vi "Valve Timer FGV.vi"(7 "Valve Timer Enum":T1, 8 "error in (no error)":errorcluster, 11 "Duration(min)":dbl) -> (0 "error out":errorcluster, 2 "Switch Valve":bool, 3 "Count Down [s]":dbl)   [LabVIEW 2020]
uses:
  controls/Valve Timer FGV.ctl
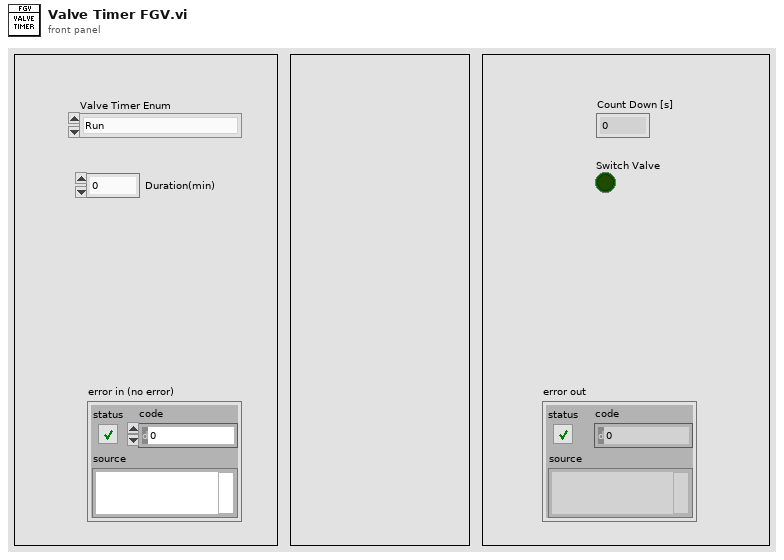
[diagram p1: front panel]
types:
  T1 = typedef "Valve Timer FGV.ctl" = enum16{"Run", "Check", "Stop"}
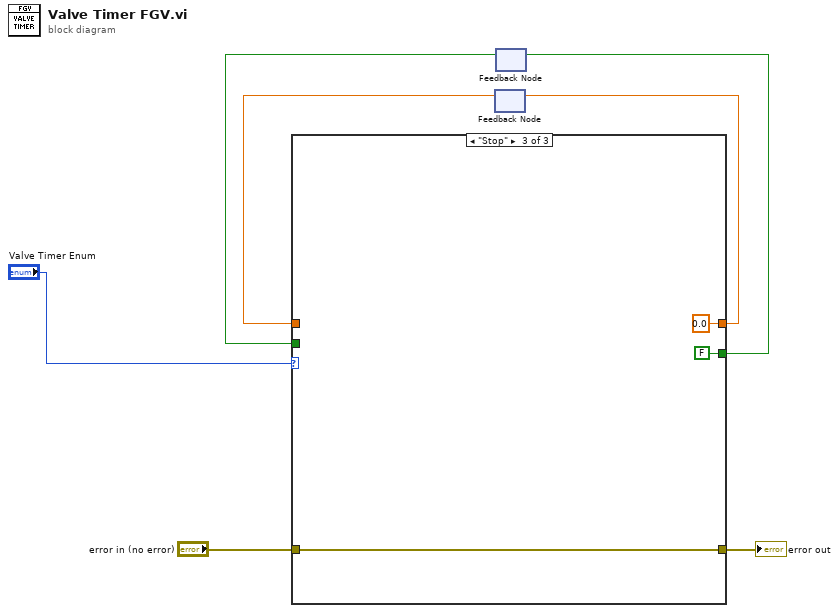
[diagram p0: block diagram]
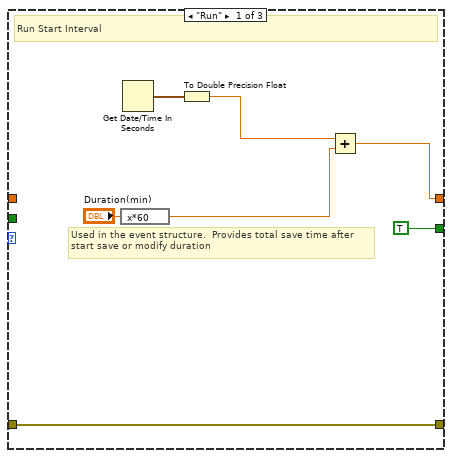
[diagram p2: hidden frame]
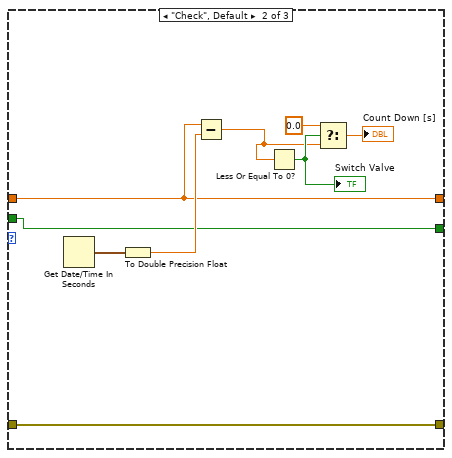
[diagram p3: hidden frame]
diagram:
  n1 = feedback #1() -> (w4:dbl)  [unwired: 1 in]
  n2 = feedback #2() -> (w1:bool)  [unwired: 1 in]
  n3 = case shown="\"Stop\"" "Valve Timer Enum" {
    tunnel: "error in (no error)" -> [w14 w23 w26]
    tunnel: [w14 w23 w26] -> w6
    tunnel: [w10 w20 0.0] -> w5
    tunnel: w4 -> [_ w20 _]
    tunnel: [TRUE w15 FALSE] -> w2
    tunnel: w1 -> [_ w15 _]
    frame "Run" {
      # "Used in the event structure.  Provides total save time after\nstart save or modify duration"
      # "Run Start Interval"
      n4 = expression code="x*60"("Duration(min)") -> (w9:dbl)
      n5 = Get Date/Time In Seconds() -> (seconds since 1Jan1904=w13:timestamp)
      n6 = To Double Precision Float(number=w13) -> (double precision float=w11:dbl)
      n7 = Add(x=w11, y=w9) -> (x+y=w10:dbl)
    }
    frame "Check", Default {
      n8 = Get Date/Time In Seconds() -> (seconds since 1Jan1904=w22:timestamp)
      n9 = To Double Precision Float(number=w22) -> (double precision float=w21:dbl)
      n10 = Subtract(x=w20, y=w21) -> (x-y=w17:dbl)
      n11 = Less Or Equal To 0?(x=w17) -> (x <= 0?=w19:bool)
      "Switch Valve" <- w19
      n12 = Select(t=0.0, s=w19, f=w17) -> (s? t:f=→"Count Down [s]":dbl)
    }
    frame "Stop" {
    }
  }
  "error out" <- w6
  n13 = feedback-in #1(w5) -> ()
  n14 = feedback-in #2(w2) -> ()
